vi "readSDOU32.vi"(6 "interface object in":refnum<k20>, 8 "error in (no error)":errorcluster, 9 "subIndex":u8, 10 "objectIndex":u16, 11 "MotorControllerClass in":refnum<class "MotorControllerClass.lvclass">) -> (0 "error out":errorcluster, 1 "interface object out":refnum<k20>, 2 "output":u32, 3 "MotorControllerClass out":refnum<class "MotorControllerClass.lvclass">)   [LabVIEW 2018, in "MotorControllerClass.lvclass"]
uses:
  BMS/MotorControllerClass.lvclass
  <vilib>/CANopenLib/CANOPEN.llb/CANopen SDO Create.vi
  <vilib>/CANopenLib/CANOPEN.llb/CANopen SDO Read [U32].vi
  <vilib>/CANopenLib/CANOPEN.llb/CANopen SDO Close.vi
panel:
  out "completion code":u32 format="%.0x"
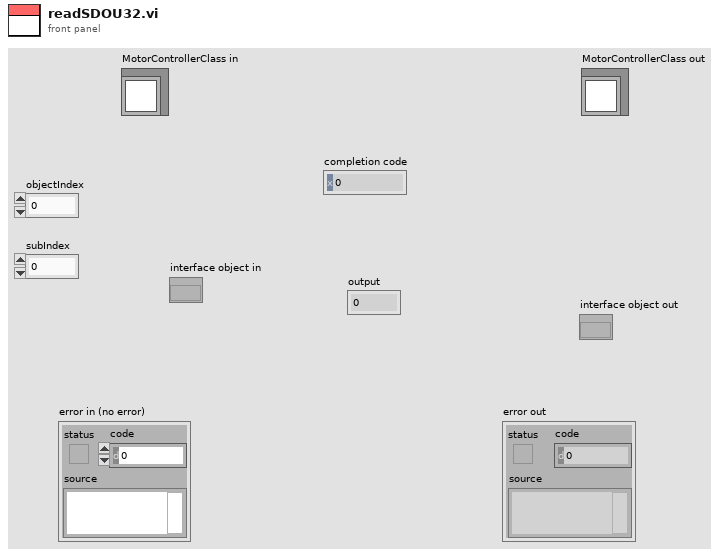
[diagram p1: front panel]
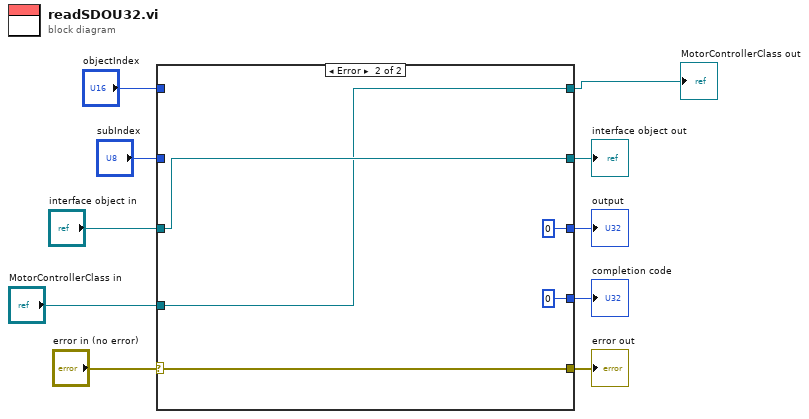
[diagram p0: block diagram]
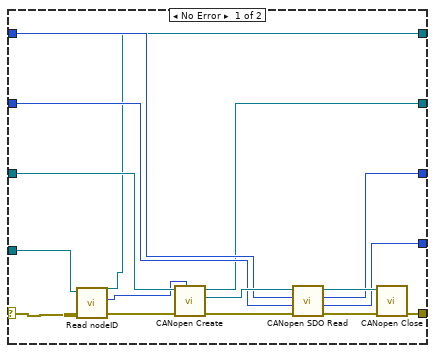
[diagram p2: hidden frame]
diagram:
  n1 = case shown="Error" "error in (no error)" {
    selector: "error in (no error)" -> [w12 w31]
    tunnel: [w18 w31] -> w8
    tunnel: [w13 w27] -> w1
    tunnel: [w22 u32 0 ("U32 data")] -> w9
    tunnel: "subIndex" -> [w21 _]
    tunnel: "objectIndex" -> [w20 _]
    tunnel: "interface object in" -> [w19 w29]
    tunnel: [w17 w29] -> w4
    tunnel: [w16 u32 0 ("completion code")] -> w3
    tunnel: "MotorControllerClass in" -> [w11 w27]
    frame No Error {
      n2 = call-dynamic "Read nodeID.vi"("error in (no error)"=w12, "MotorControllerClass in"=w11) -> ("error out"=w15:errorcluster, "nodeID"=w14:u8, "MotorControllerClass out"=w13:refnum<class "MotorControllerClass.lvclass">)  [unwired: 7 in]
      n3 = call-poly <vilib>:"CANopen Create.vi"("node-ID"=w14, "error in (no error)"=w15, "interface object in"=w19) -> ("error out"=w26:errorcluster, "SDO object out"=w25:refnum<k20>, "interface object out"=w17:refnum<k20>)  [unwired: 6 in]
      n4 = call-poly <vilib>:"CANopen SDO Read.vi"("error in (no error)"=w26, "object sub-index (0)"=w21, "object index"=w20, "SDO object in"=w25) -> ("error out"=w23:errorcluster, "completion code"=w16:u32, "U32 data"=w22:u32, "SDO object out"=w24:refnum<k20>)  [unwired: 4 in]
      n5 = call-poly <vilib>:"CANopen Close.vi"("error in (no error)"=w23, "SDO object in"=w24) -> ("error out"=w18:errorcluster)  [unwired: 9 in]
    }
    frame Error {
    }
  }
  "error out" <- w8
  "output" <- w9
  "interface object out" <- w4
  "completion code" <- w3
  "MotorControllerClass out" <- w1
